vi "Get Frames.vi"(8 "error in (no error)":errorcluster, 11 "uCAN in":refnum<class "uCAN.lvclass">) -> (0 "error out":errorcluster, 2 "readout":string, 3 "uCAN out":refnum<class "uCAN.lvclass">)   [LabVIEW 2021, in "uCanDriver.lvlib" / "uCAN.lvclass"]
uses:
  uCAN.lvclass
  uCAN.lvclass/uCAN.ctl
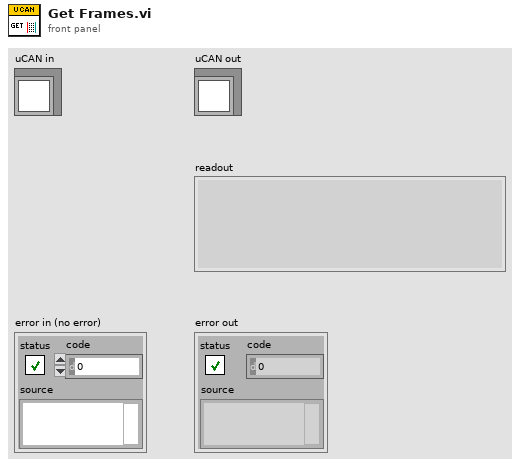
[diagram p1: front panel]
types:
  T1 = typedef "uCanDriver.lvlib/uCAN.lvclass/frame.ctl" = cluster{"Extended":bool, "ID":u32, "Data":u8[], "DLC":u8}
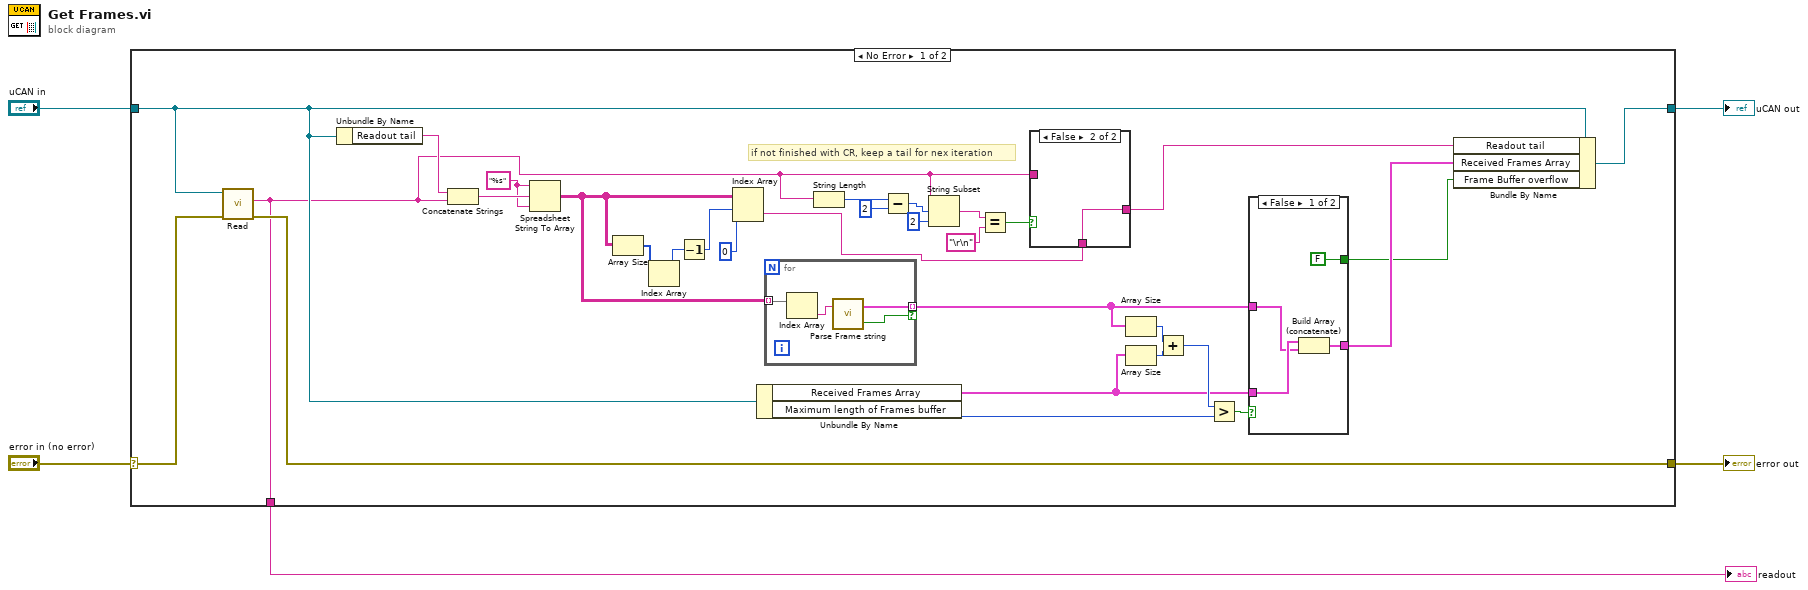
[diagram p0: block diagram]
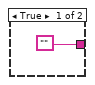
[diagram p2: hidden frame]
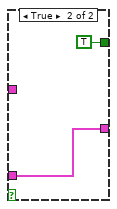
[diagram p3: hidden frame]
diagram:
  n1 = case shown="No Error" "error in (no error)" {
    selector: "error in (no error)" -> [w27 w50]
    tunnel: [w26 w50] -> w4
    tunnel: [w33 w49] -> w2
    tunnel: "uCAN in" -> [w25 w49]
    tunnel: [w6 _] -> w1
    frame No Error {
      w34 = "%s" ("format string")
      # "if not finished with CR, keep a tail for nex iteration"
      n2 = call "Read.vi"("error in (no error)"=w27, "uCAN in"=w25) -> ("error out"=w26:errorcluster, "readout"=w6:string)  [unwired: 7 in, 1 out]
      n3 = Unbundle By Name(w25) -> ("Readout tail"=w36:string)
      n4 = Concatenate Strings(w36, w6) -> (w35:string)
      n5 = Spreadsheet String To Array(format string=w34, spreadsheet string=w35, array type (2D Dbl)=w34) -> (array=w28:string[][])  [unwired: 1 in]
      n6 = Array Size(array=w28) -> (size(s)=w31:i32[])
      n7 = Index Array(array=w31) -> (element=w30:i32)  [unwired: 1 in]
      n8 = Decrement(x=w30) -> (x-1=w29:i32)
      n9 = Index Array(array=w28, index (row)=w29, index (col)=0 ("disabled index (col)")) -> (element=w7:string)
      n10 = Unbundle By Name(w25) -> ("Received Frames Array"=w19:T1[], "Maximum length of Frames buffer"=w21:i32)
      n11 = for {
        tunnel: w28 -> [w48] mode=indexing
        tunnel: [w46] -> w18 mode=indexing if=w45
        n12 = Index Array(array=w48) -> (element=w47:string)  [unwired: 1 in]
        n13 = call "Parse Frame string.vi"("frame string"=w47) -> ("Parse OK"=w45:bool, "output cluster"=w46:T1)  [unwired: 1 in]
      }
      n14 = String Length(string=w6) -> (length=w15:i32)
      n15 = Subtract(x=w15, y=2) -> (x-y=w13:i32)
      n16 = String Subset(string=w6, offset (0)=w13, length (rest)=2 ("length (rest)")) -> (substring=w11:string)
      n17 = Equal?(x=w11, y="\r\n") -> (x = y?=w9:bool)
      n18 = case shown="False" w9 {
        tunnel: ["" w38] -> w8
        tunnel: w6 -> [_ _]
        tunnel: w7 -> [_ w38]
        frame True {
        }
        frame False {
        }
      }
      n19 = Array Size(array=w18) -> (size(s)=w24:i32)
      n20 = Array Size(array=w19) -> (size(s)=w23:i32)
      n21 = Add(x=w24, y=w23) -> (x+y=w22:i32)
      n22 = Greater?(x=w22, y=w21) -> (0:w20:bool)
      n23 = case shown="False" w20 {
        tunnel: w19 -> [w42 w44]
        tunnel: w18 -> [w41 _]
        tunnel: [w40 w44] -> w17
        tunnel: [FALSE TRUE] -> w16
        frame False {
          n24 = Build Array (concatenate)(w42, w41) -> (w40:T1[])
        }
        frame True {
        }
      }
      n25 = Bundle By Name(cluster=w25, "Readout tail"=w8, "Received Frames Array"=w17, "Frame Buffer overflow"=w16) -> (w33:refnum<class "uCAN.lvclass">)
    }
    frame Error {
    }
  }
  "error out" <- w4
  "uCAN out" <- w2
  "readout" <- w1
